vi "Mark Read Only.vi"(8 "error in (no error)":errorcluster, 11 "Promise in":refnum<class "Promise.lvclass">) -> (0 "error out":errorcluster, 3 "Promise out":refnum<class "Promise.lvclass">)   [LabVIEW 2020, in "Promises.lvlib" / "Promise.lvclass"]
doc: "Prevents the Promise value returned from the VI to be used for resolving the Promise. This is useful when the Promise is created within a subVI and passed along to a task and preventing the caller from incorrectly using the Promise since only the task should be calling <b>Resolve</b>. The returned Promise value can still be used to send a parameter to the task."
uses:
  Promise.lvclass
  Promise.lvclass/Promise.ctl
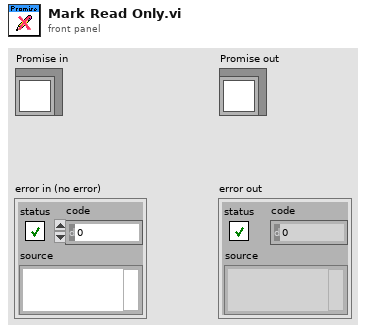
[diagram p1: front panel]
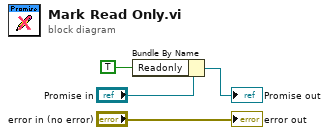
[diagram p0: block diagram]
diagram:
  n1 = Bundle By Name(cluster="Promise in", "Readonly"=TRUE) -> (→"Promise out":refnum<class "Promise.lvclass">)
  "error out" <- "error in (no error)"
